vi "LSX Set Controller.vi"(6 "lAC":i32, 7 "lZC":i32, 8 "error in (no error)":errorcluster, 9 "lYC":i32, 10 "lXC":i32, 11 "lLSID":i32) -> (0 "error out":errorcluster, 3 "function return":i32)   [LabVIEW 2018, in "Tango.lvlib"]
doc: "TANGOAPI int TANGOCALL LSX_SetController (int lLSID, int lXC, int lYC, int lZC, int lAC);"
uses:
  Tango.lvlib
  SubVIs/Tango_DLL.dll
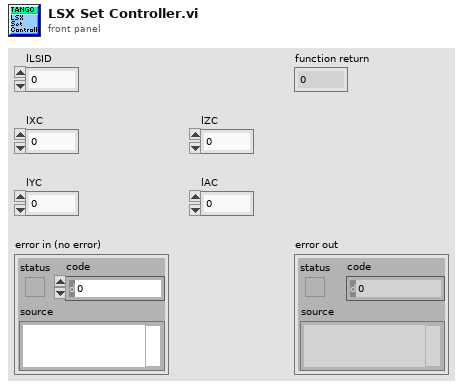
[diagram p1: front panel]
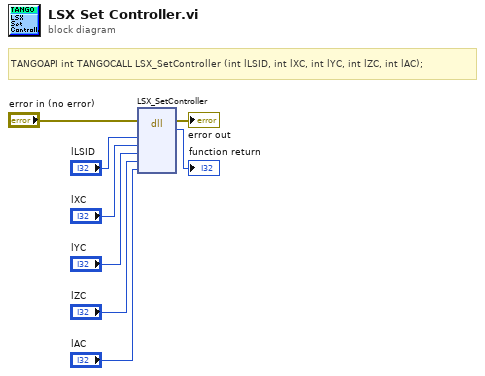
[diagram p0: block diagram]
diagram:
  # "TANGOAPI int TANGOCALL LSX_SetController (int lLSID, int lXC, int lYC, int lZC, int lAC);"
  n1 = dll-call lib="C:/Users/Familie/Documents/LabviewIX81/lib/TANGO Stage/SubVIs/Tango_DLL.*" fn="LSX_SetController"(error in="error in (no error)", "lLSID"="lLSID", "lXC"="lXC", "lYC"="lYC", "lZC"="lZC", "lAC"="lAC") -> (error out=→"error out":errorcluster, →"function return":i32)  [unwired: 7 in, 1 out]
